vi "AlliGator Check HDF5 File Type.vi"(8 "error in (no error)":errorcluster, 11 "HDF5 File Path in":path) -> (0 "error out":errorcluster, 1 "FLI Dataset?":bool, 2 "FLI Dataset Type":T1, 3 "HDF5 File Path out":path)   [LabVIEW 2021, in "AlliGator HDF5.lvlib"]
doc: "Tries reading the HDF5 file's information for the 3 different supported dataset type, until success, and returns the identified dataset type."
uses:
  AlliGator HDF5.lvlib
  AlliGator FLI Dataset Type.ctl
  <vilib>/Utility/error.llb/Error Cluster From Error Code.vi
  <vilib>/ErrorRing/Error Ring.xnode
  AlliGator Files.lvlib
  SwissSPAD/SwissSPAD.lvlib
panel:
  # "see the AlliGator License on the block diagram (Ctrl+E or Window:Show Block Diagram)"
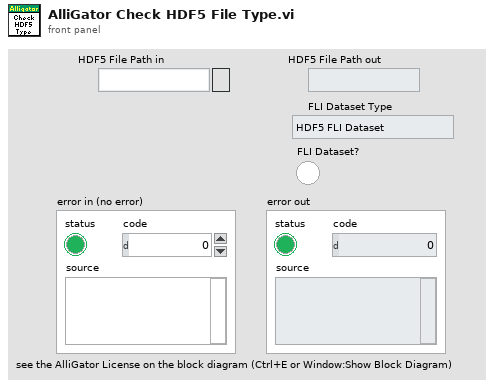
[diagram p1: front panel]
types:
  T1 = typedef "AlliGator Files.lvlib/AlliGator FLI Dataset Type.ctl" = enum16{"HDF5 FLI Dataset", "Gate Image Folder", ".sdt FLI Dataset (Becker & Hickl)", ".ptu FLI Dataset (PicoQuant)", "SS1 FLI Dataset", "SS2 FLI Dataset", "I/m/phi Dataset", ".bin FLI Dataset (PicoQuant Binned)", ".bin FLI Dataset (Piccolo Binned)"}
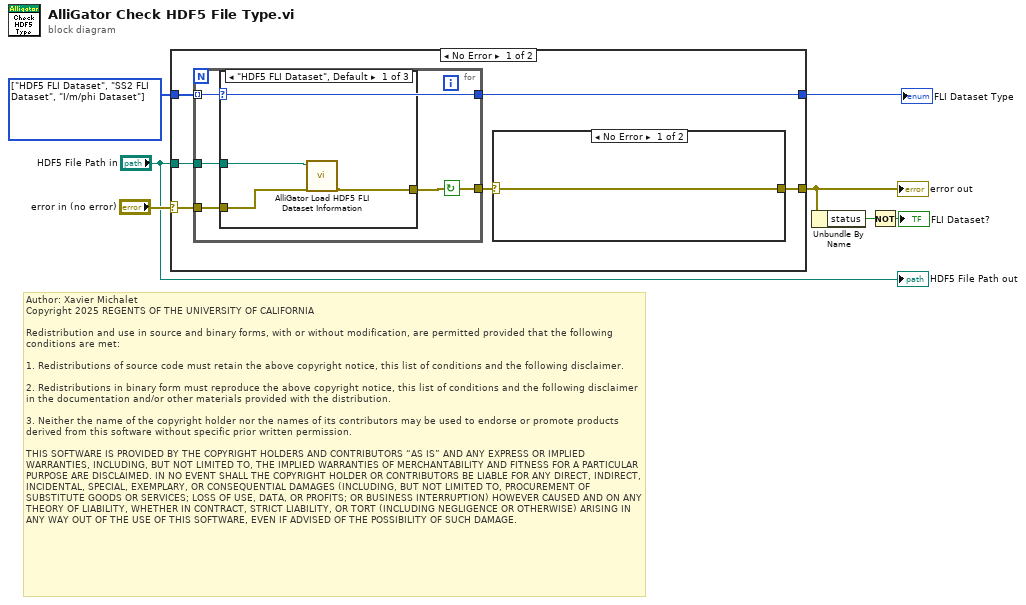
[diagram p0: block diagram]
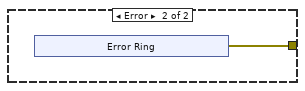
[diagram p2: hidden frame]
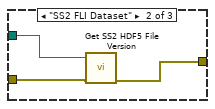
[diagram p3: hidden frame]
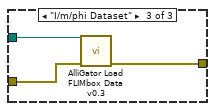
[diagram p4: hidden frame]
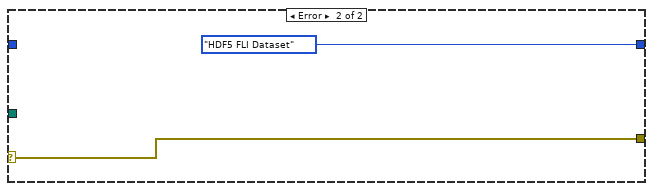
[diagram p5: hidden frame]
diagram:
  w7 = T1[] [enum."HDF5 FLI Dataset", enum."SS2 FLI Dataset", enum."I/m/phi Dataset"] items=["HDF5 FLI Dataset", "Gate Image Folder", ".sdt FLI Dataset (Becker & Hickl)", ".ptu FLI Dataset (PicoQuant)", "SS1 FLI Dataset", "SS2 FLI Dataset", "I/m/phi Dataset", ".bin FLI Dataset (PicoQuant Binned)", ".bin FLI Dataset (Piccolo Binned)"] ("Array")
  # "Author: Xavier Michalet\nCopyright 2025 REGENTS OF THE UNIVERSITY OF CALIFORNIA\n\nRedistribution and use in source and binary forms, with or without modification, are permitted provided that the following conditions are met:\n\n1. Redistributions of source code must retain the above copyright notice, this list of conditions and the following disclaimer.\n\n2. Redistributions in binary form must reproduce the above copyright notice, this list of conditions and the following disclaimer in the documentation and/or other materials provided with the distribution.\n\n3. Neither the name of the copyright holder nor the names of its contributors may be used to endorse or promote products derived from this software without specific prior written permission.\n\nTHIS SOFTWARE IS PROVIDED BY THE COPYRIGHT HOLDERS AND CONTRIBUTORS “AS IS” AND ANY EXPRESS OR IMPLIED WARRANTIES, INCLUDING, BUT NOT LIMITED TO, THE IMPLIED WARRANTIES OF MERCHANTABILITY AND FITNESS FOR A PARTICULAR PURPOSE ARE DISCLAIMED. IN NO EVENT SHALL THE COPYRIGHT HOLDER OR CONTRIBUTORS BE LIABLE FOR ANY DIRECT, INDIRECT, INCIDENTAL, SPECIAL, EXEMPLARY, OR CONSEQUENTIAL DAMAGES (INCLUDING, BUT NOT LIMITED TO, PROCUREMENT OF SUBSTITUTE GOODS OR SERVICES; LOSS OF USE, DATA, OR PROFITS; OR BUSINESS INTERRUPTION) HOWEVER CAUSED AND ON ANY THEORY OF LIABILITY, WHETHER IN CONTRACT, STRICT LIABILITY, OR TORT (INCLUDING NEGLIGENCE OR OTHERWISE) ARISING IN ANY WAY OUT OF THE USE OF THIS SOFTWARE, EVEN IF ADVISED OF THE POSSIBILITY OF SUCH DAMAGE."
  n1 = case shown="No Error" "error in (no error)" {
    selector: "error in (no error)" -> [w11 w33]
    tunnel: w7 -> [w13 _]
    tunnel: "HDF5 File Path in" -> [w12 _]
    tunnel: [w8 w33] -> w3
    tunnel: [w10 AlliGator_FLI_Dataset_Type."HDF5 FLI Dataset" ("FLI Dataset Type")] -> w5
    frame No Error {
      n2 = for {
        tunnel: w13 -> [w20] mode=indexing
        tunnel: w12 -> [w23]
        tunnel: w11 -> [w22]
        tunnel: [w21] -> w9
        tunnel: [w20] -> w10
        stop <- w21 continue-if-true
        n3 = case shown="\"HDF5 FLI Dataset\", Default" w20 {
          tunnel: w23 -> [w26 w28 w32]
          tunnel: w22 -> [w25 w29 w31]
          tunnel: [w24 w27 w30] -> w21
          frame "HDF5 FLI Dataset", Default {
            n4 = call "AlliGator Load HDF5 FLI Dataset Information.vi"("Error In"=w25, "File Path"=w26) -> ("error out"=w24:errorcluster)  [unwired: 5 in, 4 out]
          }
          frame "SS2 FLI Dataset" {
            n5 = call "Get SS2 HDF5 File Version.vi"("error in (no error)"=w29, "path in"=w28) -> ("error out"=w27:errorcluster)  [unwired: 7 in, 2 out]
          }
          frame "I/m/phi Dataset" {
            n6 = call "AlliGator Load FLIMbox Data v0.3.vi"("Error In"=w31, "File Path"=w32) -> ("Error Out"=w30:errorcluster)  [unwired: 8 in, 1 out]
          }
        }
      }
      n7 = case shown="No Error" w9 {
        selector: w9 -> [w14 _]
        tunnel: [w14 w15] -> w8
        frame No Error {
        }
        frame Error {
          n8 = xnode "Error Ring"() -> ("error out"=w15:errorcluster)
        }
      }
    }
    frame Error {
    }
  }
  "error out" <- w3
  "FLI Dataset Type" <- w5
  n9 = Unbundle By Name(w3) -> ("status"=w2:bool)
  n10 = Not(x=w2) -> (.not. x?=→"FLI Dataset?":bool)
  "HDF5 File Path out" <- "HDF5 File Path in"
